vi "FGV_DVR.vi"(7 "Set":bool, 8 "error in (no error)":errorcluster caption="错误输入（无错误）", 11 "DVR":refnum<data-value>) -> (0 "error out":errorcluster caption="错误输出", 3 "DVR":refnum<data-value>)   [LabVIEW 2011, in "CAN FD.lvlib"]
uses:
  CAN FD.lvlib
  Typedef/CAN Data.ctl
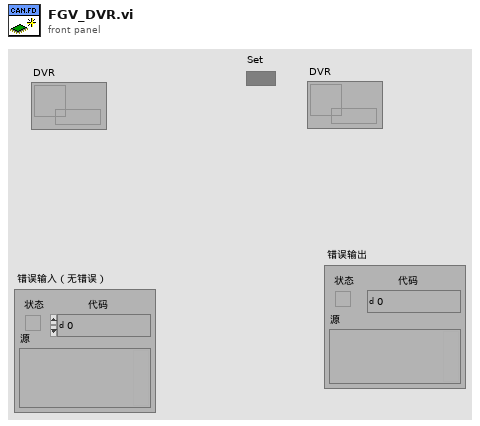
[diagram p1: front panel]
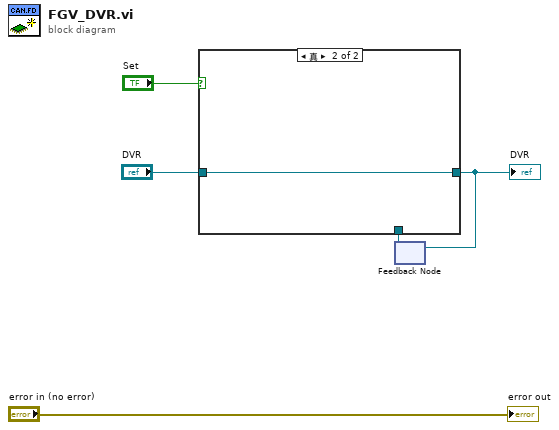
[diagram p0: block diagram]
diagram:
  n1 = feedback #1() -> (w1:refnum<data-value>)  [unwired: 1 in]
  n2 = case shown="真" "Set" {
    tunnel: "DVR" -> [_ w7]
    tunnel: [w6 w7] -> w2
    tunnel: w1 -> [w6 _]
    frame False {
    }
    frame True {
    }
  }
  "DVR" <- w2
  n3 = feedback-in #1(w2) -> ()
  "error out" <- "error in (no error)"
